vi "ArraySelect.vi"(8 "Winch Pot":dbl) -> (0 "Button Pressed":bool, 3 "Winch Location":dbl)   [LabVIEW 2013]
panel:
  in  "three":bool
  in  "two":bool
  in  "one":bool
  in  "Array":dbl[](array[numeric])
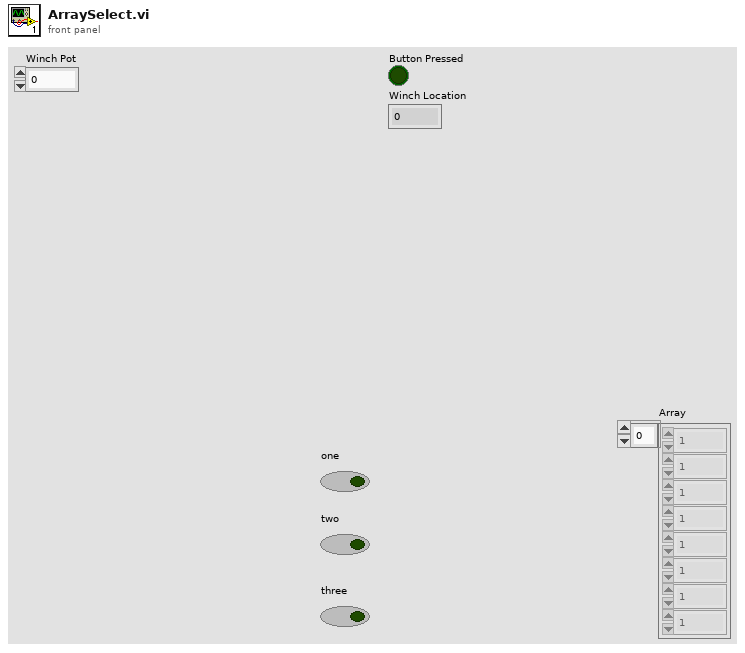
[diagram p1: front panel]
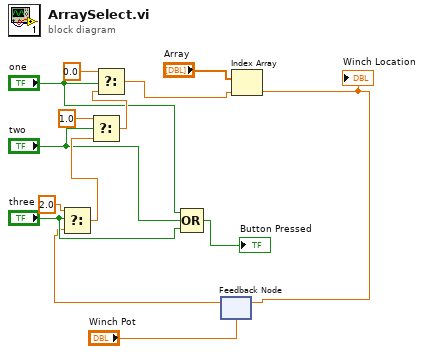
[diagram p0: block diagram]
diagram:
  n1 = Compound Arithmetic op=OR("one", "two", "three") -> (→"Button Pressed":bool)
  n2 = feedback #1("Winch Pot") -> (w2:dbl)
  n3 = Select(t=2.0, s="three", f=w2) -> (s? t:f=w14:dbl)
  n4 = Select(t=1.0, s="two", f=w14) -> (s? t:f=w13:dbl)
  n5 = Select(t=0.0, s="one", f=w13) -> (s? t:f=w4:dbl)
  n6 = Index Array(array="Array", index=w4) -> (element=w3:dbl)
  "Winch Location" <- w3
  n7 = feedback-in #1(w3) -> ()
